vi "HEWH Start PID Conditions.vi"(4 "Disable Purge":bool, 6 "State":T1, 8 "Error In":errorcluster, 9 "TC Down":dbl, 11 "Elapsed Time (sec)":dbl) -> (0 "Error Out":errorcluster, 3 "Adjusting Temp":bool)   [LabVIEW 2019]
uses:
  Type Definitions/HEWH Purge Draw.ctl
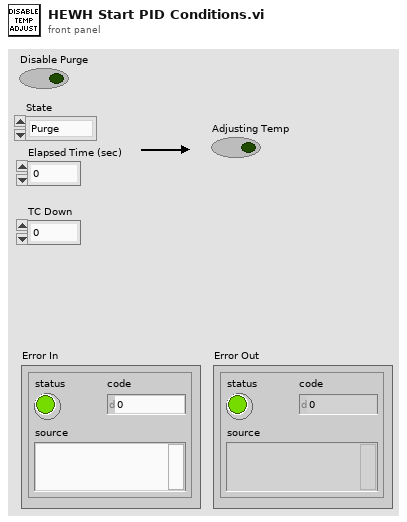
[diagram p1: front panel]
types:
  T1 = typedef "HEWH Purge Draw.ctl" = enum16{"Purge", "Draw"}
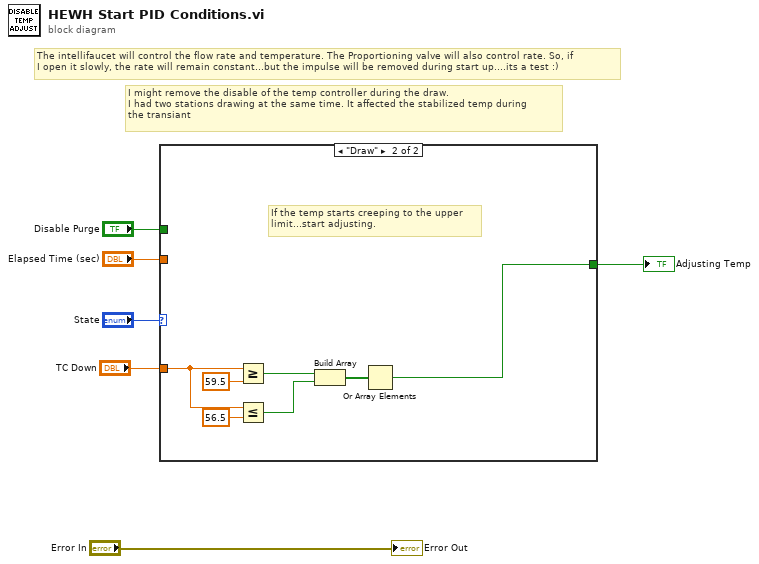
[diagram p0: block diagram]
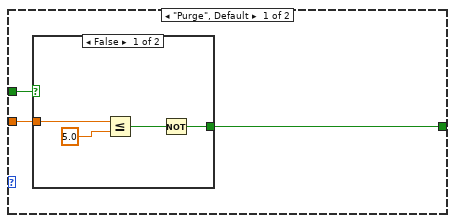
[diagram p2: hidden frame]
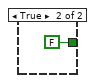
[diagram p3: hidden frame]
diagram:
  # "I might remove the disable of the temp controller during the draw.\nI had two stations drawing at the same time. It affected the stabilized temp during \nthe transiant"
  # "The intellifaucet will control the flow rate and temperature. The Proportioning valve will also control rate. So, if \nI open it slowly, the rate will remain constant...but the impulse will be removed during start up....its a test :)"
  n1 = case shown="\"Draw\"" "State" {
    tunnel: "Elapsed Time (sec)" -> [w9 _]
    tunnel: [w8 w15] -> w3
    tunnel: "Disable Purge" -> [w7 _]
    tunnel: "TC Down" -> [_ w19]
    frame "Purge", Default {
      n2 = case shown="False" w7 {
        tunnel: w9 -> [w12 _]
        tunnel: [w10 FALSE] -> w8
        frame False {
          n3 = Less Or Equal?(x=w12, y=5.0) -> (x <= y?=w11:bool)
          n4 = Not(x=w11) -> (.not. x?=w10:bool)
        }
        frame True {
        }
      }
    }
    frame "Draw" {
      # "If the temp starts creeping to the upper \nlimit...start adjusting."
      n5 = Greater Or Equal?(x=w19, y=59.5) -> (x >= y?=w18:bool)
      n6 = Less Or Equal?(x=w19, y=56.5) -> (x <= y?=w17:bool)
      n7 = Build Array(w18, w17) -> (w16:bool[])
      n8 = Or Array Elements(Boolean array=w16) -> (logical OR=w15:bool)
    }
  }
  "Adjusting Temp" <- w3
  "Error Out" <- "Error In"
